vi "Set All CD Item Property Values.vi"(8 "error in (no error)":errorcluster, 11 "CD Parameter Manager in":refnum<class "CD Parameter Manager.lvclass">) -> (0 "error out":errorcluster, 3 "CD Parameter Manager out":refnum<class "CD Parameter Manager.lvclass">)   [LabVIEW 2019, in "CD Parameter Manager API.lvlib" / "CD Parameter Manager.lvclass"]
uses:
  CD Parameter Manager.lvclass
  CD Parameter Manager.lvclass/CD Parameter Manager.ctl
  Parameter Class/Parameter.lvclass
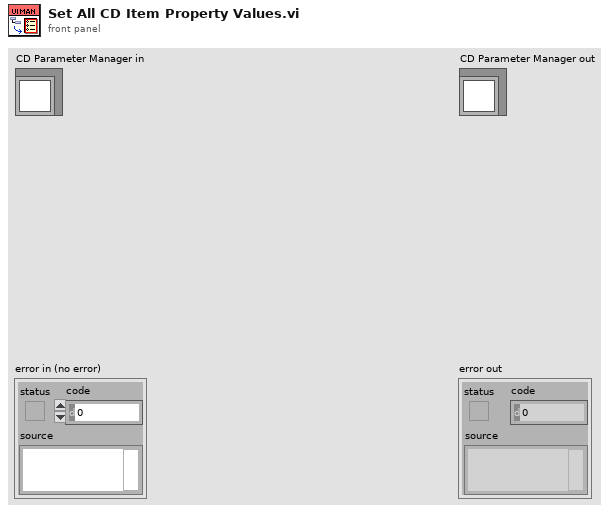
[diagram p1: front panel]
types:
  T1 = cluster{"Group name":string, "Controls":refnum<class "Parameter.lvclass">[]}[]
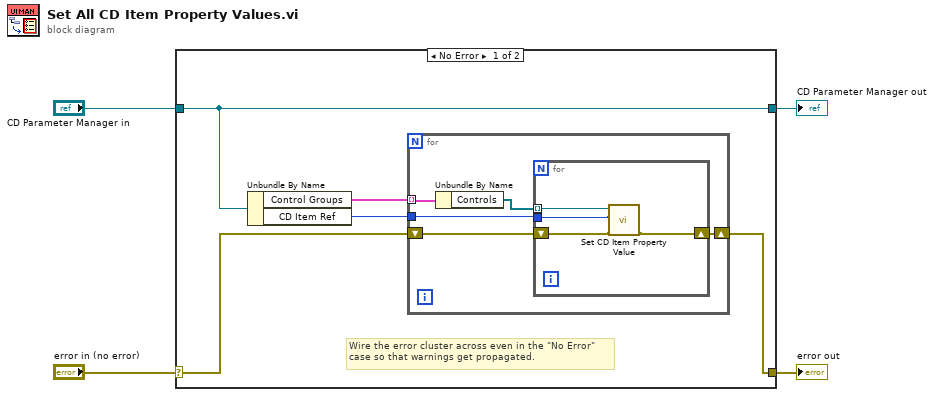
[diagram p0: block diagram]
diagram:
  n1 = case shown="No Error" "error in (no error)" {
    selector: "error in (no error)" -> [w6 w20]
    tunnel: [w5 w20] -> w3
    tunnel: [w7 w19] -> w1
    tunnel: "CD Parameter Manager in" -> [w7 w19]
    frame No Error {
      # "Wire the error cluster across even in the \"No Error\"\ncase so that warnings get propagated."
      n2 = Unbundle By Name(w7) -> ("Control Groups"=w9:T1, "CD Item Ref"=w8:u64)
      n3 = for {
        tunnel: w9 -> [w11] mode=indexing
        tunnel: w8 -> [w14]
        shift-right: [w12] -> w5
        shift-left: w6 -> [w13]
        n4 = Unbundle By Name(w11) -> ("Controls"=w10:refnum<class "Parameter.lvclass">[])
        n5 = for {
          tunnel: w14 -> [w16]
          shift-right: [w17] -> w12
          shift-left: w13 -> [w18]
          tunnel: w10 -> [w15] mode=indexing
          n6 = call-dynamic "Set CD Item Property Value.vi"("error in (no error)"=w18, "CD Item Ref in"=w16, "Parameter in"=w15) -> ("error out"=w17:errorcluster)  [unwired: 7 in, 1 out]
        }
      }
    }
    frame Error {
    }
  }
  "error out" <- w3
  "CD Parameter Manager out" <- w1
